vi "Proyecto.vi"() -> ()   [LabVIEW 2020]
uses:
  <vilib>/Utility/error.llb/DialogType.ctl
  <vilib>/Instr/_visa.llb/VISA Configure Serial Port (Instr).vi
panel:
  out "error out 2":errorcluster
  out "error out":errorcluster
  out "x+y":dbl
  out "Shape":i32
  out "B":i32
  out "G":i32
  out "R":i32
  out "Green object":dbl
  in  "ESP":bool
  in  "MATLAB":bool
  out "Position":i32
  out "Shape":picture
  out "Blue object":dbl
  out "Red object":dbl
  out "Color":u32(colorbox)
  out "Object presence":i32
  in  "Speed Control":dbl(slide) scale=80.0..100.0
  out "Band speed":dbl(knob) scale=0.0..10.0
  in  "ESP port":refnum<visa-resource-name>
  in  "Matlab port":refnum<visa-resource-name>
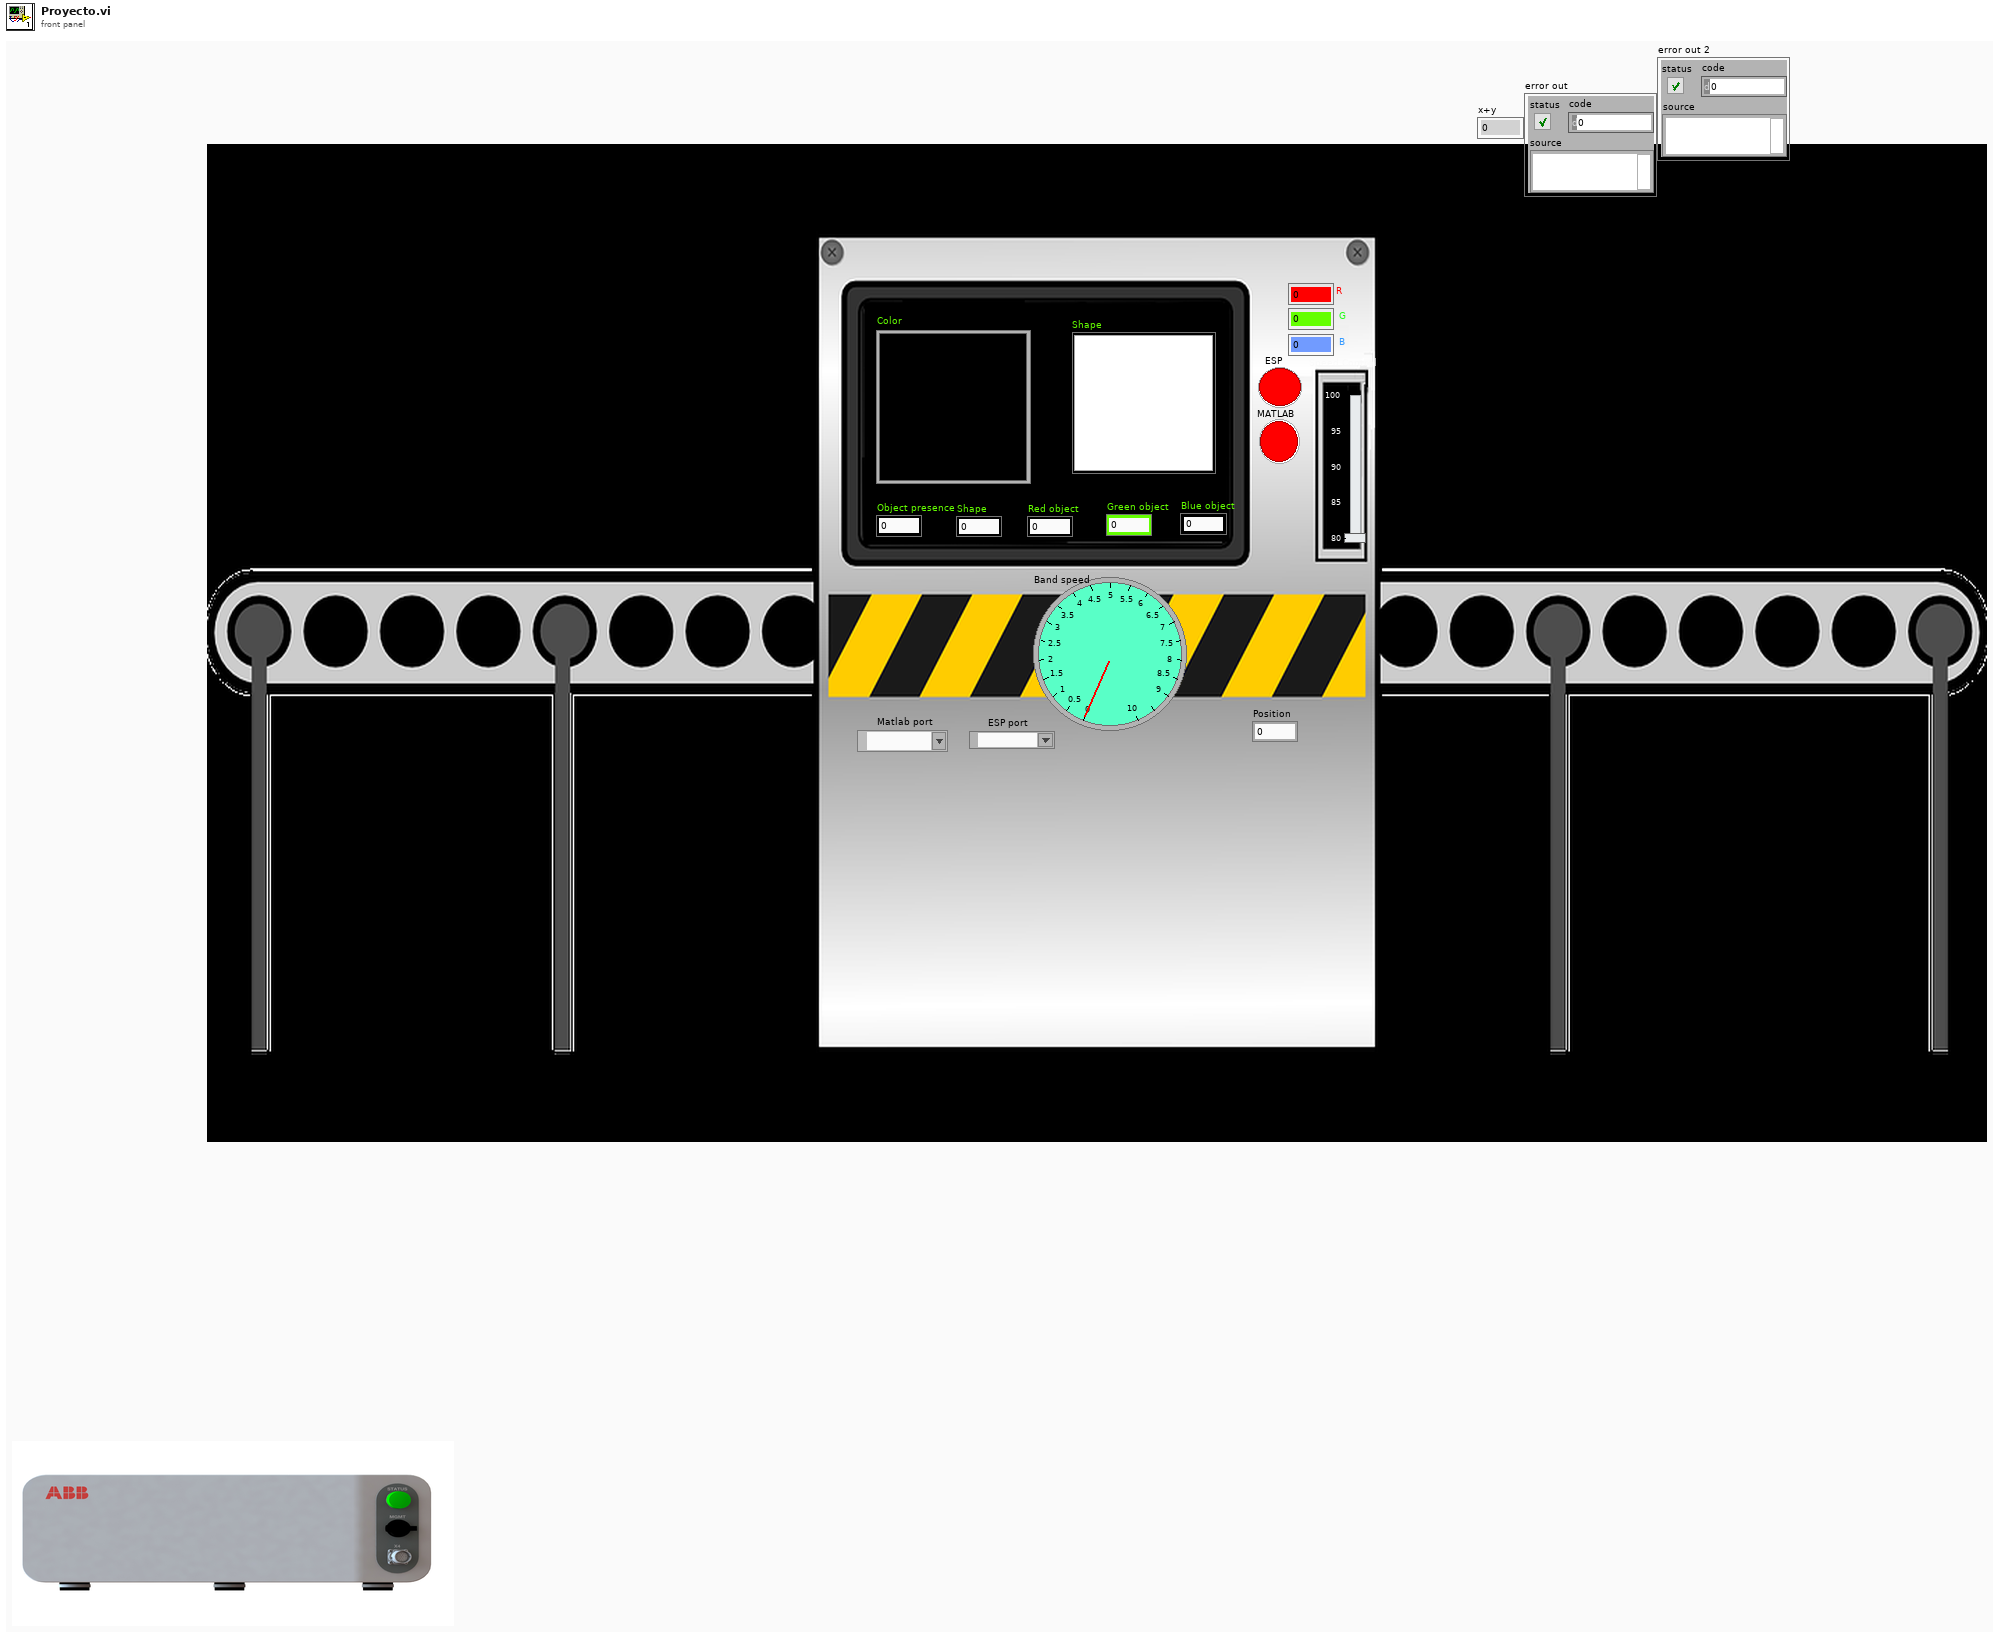
[diagram p1: front panel]
types:
  T1 = typedef "DialogType.ctl" = u16
  T2 = typedef "imagedata.ctl" = cluster{"image type":i32, "image depth":i32, "image":u8[], "mask":u8[], "colors":u32[], "Rectangle":cluster{"left":i16, "top":i16, "right":i16, "bottom":i16}}
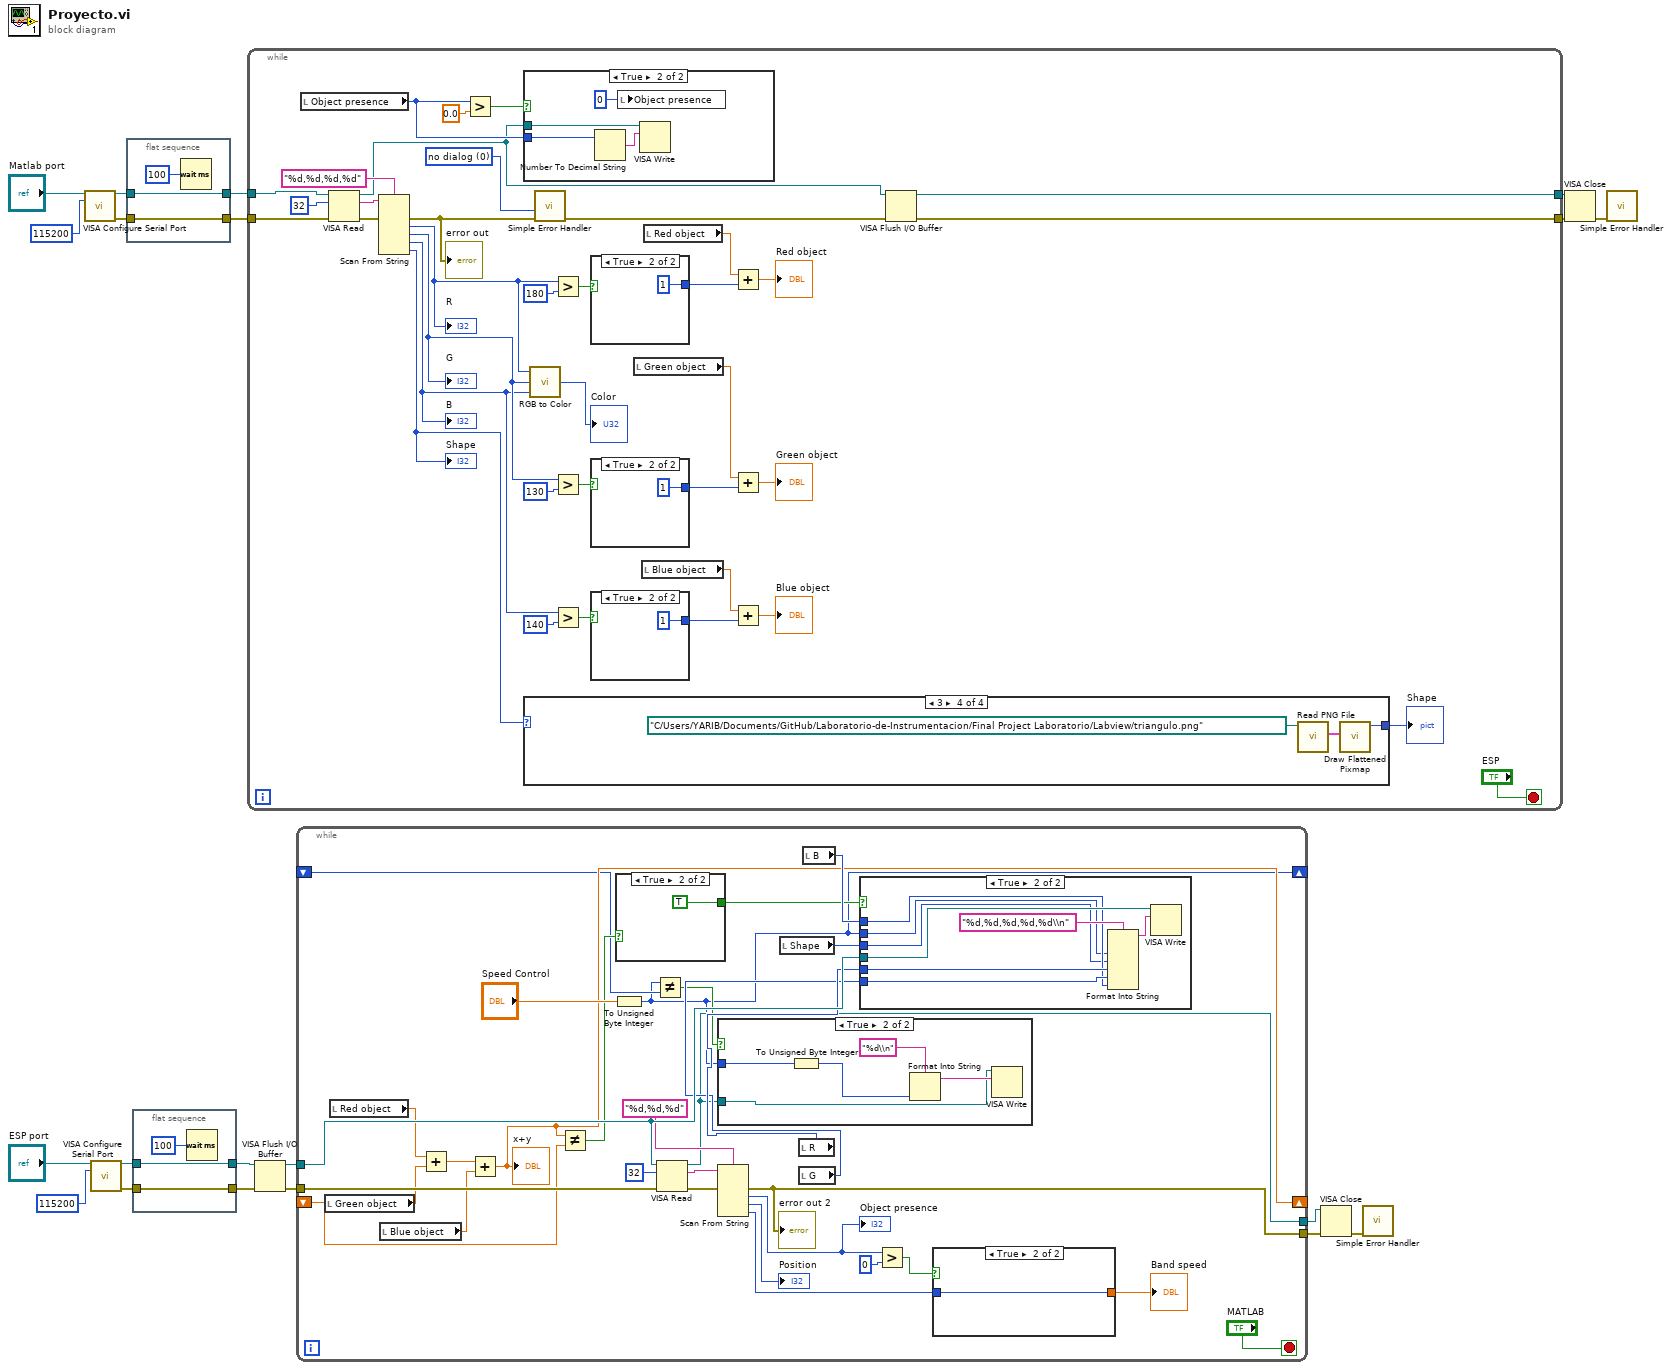
[diagram p0: block diagram]
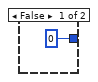
[diagram p2: hidden frame]
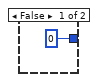
[diagram p4: hidden frame]
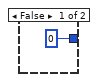
[diagram p5: hidden frame]
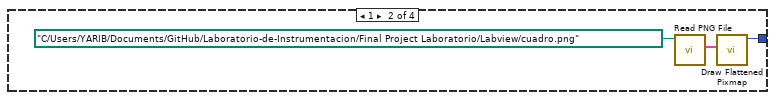
[diagram p7: hidden frame]
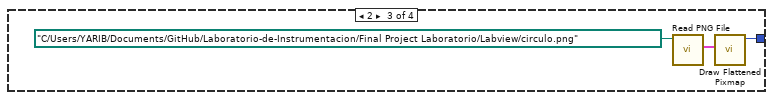
[diagram p8: hidden frame]
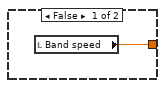
[diagram p9: hidden frame]
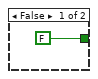
[diagram p11: hidden frame]
diagram:
  n1 = call-poly "VISA Configure Serial Port"("VISA resource name"="Matlab port", "baud rate (9600)"=u32 115200) -> ("VISA resource name out"=w10:refnum<visa-resource-name>, "error out"=w9:errorcluster)  [unwired: 12 in]
  n2 = call-poly "VISA Configure Serial Port"("VISA resource name"="ESP port", "baud rate (9600)"=u32 115200) -> ("VISA resource name out"=w3:refnum<visa-resource-name>, "error out"=w2:errorcluster)  [unwired: 12 in]
  n3 = flat-sequence {
    tunnel: w10 -> [w23]
    tunnel: [w23] -> w8
    tunnel: w9 -> [w22]
    tunnel: [w22] -> w7
    frame #0 {
      n4 = Wait (ms)(milliseconds to wait=u32 100) -> ()  [unwired: 1 out]
    }
  }
  n5 = flat-sequence {
    tunnel: w3 -> [w26]
    tunnel: w2 -> [w24]
    tunnel: [w26] -> w6
    tunnel: [w24] -> w1
    frame #0 {
      n6 = Wait (ms)(milliseconds to wait=u32 100) -> ()  [unwired: 1 out]
    }
  }
  n7 = while {
    tunnel: [w27] -> w13
    tunnel: [w28] -> w12
    tunnel: w8 -> [w33]
    tunnel: w7 -> [w32]
    stop <- "ESP" stop-if-true
    w54 = T1 0 items=["no dialog", "OK message", "continue or stop message", "OK message + warnings", "continue/stop + warnings"] ("type of dialog (OK msg:1)")
    n8 = local read "Object presence"() -> (w34:i32)
    n9 = VISA Read(VISA resource name=w33, byte count=u32 32, error in (no error)=w32) -> (VISA resource name out=w30:refnum<visa-resource-name>, read buffer=w56:string, error out=w57:errorcluster)  [unwired: 1 out]
    n10 = Scan From String(format string="%d,%d,%d,%d", input string=w56, error in=w57) -> (error out=w55:errorcluster, output 1=w46:i32, output 2=w48:i32, output 3=w47:i32, output 4=w49:i32)  [unwired: 5 in, 2 out]
    "R" <- w46
    "G" <- w48
    "B" <- w47
    "Shape" <- w49
    "error out" <- w55
    n11 = Greater?(x=w34, y=0.0) -> (0:w36:bool)
    n12 = case shown="True" w36 {
      tunnel: w30 -> [_ w69]
      tunnel: w34 -> [_ w68]
      frame False {
      }
      frame True {
        n13 = Number To Decimal String(number=w68) -> (decimal integer string=w67:string)  [unwired: 1 in]
        n14 = local write "Object presence"(0 ("Object presence")) -> ()
        n15 = VISA Write(VISA resource name=w69, write buffer=w67) -> ()  [unwired: 1 in, 3 out]
      }
    }
    n16 = case shown="3" w49 {
      tunnel: [_ w75 w78 w81] -> w60
      frame 0, Default {
      }
      frame 1 {
        n17 = call <vilib>:"Read PNG File.vi"("path to PNG file"=path "C:/Users/YARIB/Documents/GitHub/Laboratorio-de-Instrumentacion/Final Project Laboratorio/Labview/cuadro.png") -> ("image data"=w76:T2)  [unwired: 8 in, 2 out]
        n18 = call <vilib>:"Draw Flattened Pixmap.vi"("image data"=w76) -> ("new picture"=w75:picture)  [unwired: 8 in]
      }
      frame 2 {
        n19 = call <vilib>:"Read PNG File.vi"("path to PNG file"=path "C:/Users/YARIB/Documents/GitHub/Laboratorio-de-Instrumentacion/Final Project Laboratorio/Labview/circulo.png") -> ("image data"=w79:T2)  [unwired: 8 in, 2 out]
        n20 = call <vilib>:"Draw Flattened Pixmap.vi"("image data"=w79) -> ("new picture"=w78:picture)  [unwired: 8 in]
      }
      frame 3 {
        n21 = call <vilib>:"Read PNG File.vi"("path to PNG file"=path "C:/Users/YARIB/Documents/GitHub/Laboratorio-de-Instrumentacion/Final Project Laboratorio/Labview/triangulo.png") -> ("image data"=w82:T2)  [unwired: 8 in, 2 out]
        n22 = call <vilib>:"Draw Flattened Pixmap.vi"("image data"=w82) -> ("new picture"=w81:picture)  [unwired: 8 in]
      }
    }
    "Shape" <- w60
    n23 = call <vilib>:"RGB to Color.vi"("B"=w47, "G"=w48, "R"=w46) -> ("Color"=→"Color":u32)
    n24 = call <vilib>:"Simple Error Handler.vi"("type of dialog (OK msg:1)"=w54, "error in (no error)"=w55) -> ("error out"=w29:errorcluster)  [unwired: 3 in, 4 out]
    n25 = Greater?(x=w46, y=180) -> (0:w62:bool)
    n26 = Greater?(x=w48, y=130) -> (0:w53:bool)
    n27 = Greater?(x=w47, y=140) -> (0:w61:bool)
    n28 = case shown="True" w62 {
      tunnel: [0 1 ("y")] -> w42
      frame False {
      }
      frame True {
      }
    }
    n29 = case shown="True" w53 {
      tunnel: [0 1 ("y")] -> w45
      frame False {
      }
      frame True {
      }
    }
    n30 = case shown="True" w61 {
      tunnel: [0 1 ("y")] -> w39
      frame False {
      }
      frame True {
      }
    }
    n31 = local read "Green object"() -> (w43:dbl)
    n32 = local read "Blue object"() -> (w37:dbl)
    n33 = local read "Red object"() -> (w40:dbl)
    n34 = Add(x=w40, y=w42) -> (x+y=→"Red object":dbl)
    n35 = Add(x=w43, y=w45) -> (x+y=→"Green object":dbl)
    n36 = Add(x=w37, y=w39) -> (x+y=→"Blue object":dbl)
    n37 = VISA Flush I/O Buffer(VISA resource name=w30, error in (no error)=w29) -> (VISA resource name out=w27:refnum<visa-resource-name>, error out=w28:errorcluster)  [unwired: 1 in]
  }
  n38 = VISA Flush I/O Buffer(VISA resource name=w6, error in (no error)=w1) -> (VISA resource name out=w5:refnum<visa-resource-name>, error out=w4:errorcluster)  [unwired: 1 in]
  n39 = while {
    tunnel: w5 -> [w112]
    tunnel: [w90] -> w16
    tunnel: w4 -> [w113]
    tunnel: [w111] -> w17
    shift-right: [w94] -> _
    shift-left: _ -> [w93]
    shift-right: [w88] -> _
    shift-left: _ -> [w89]
    stop <- "MATLAB" stop-if-true
    n40 = local read "Green object"() -> (w100:dbl)
    n41 = local read "Red object"() -> (w99:dbl)
    n42 = local read "Blue object"() -> (w98:dbl)
    n43 = Add(x=w99, y=w100) -> (x+y=w101:dbl)
    n44 = Add(x=w101, y=w98) -> (x+y=w94:dbl)
    "x+y" <- w94
    n45 = Not Equal?(x=w94, y=w93) -> (x != y?=w95:bool)
    n46 = To Unsigned Byte Integer(number="Speed Control") -> (unsigned 8bit integer=w88:u8)
    n47 = case shown="True" w95 {
      tunnel: [FALSE TRUE] -> w97
      frame False {
      }
      frame True {
      }
    }
    n48 = Not Equal?(x=w88, y=w89) -> (x != y?=w91:bool)
    n49 = VISA Read(VISA resource name=w112, byte count=u32 32, error in (no error)=w113) -> (VISA resource name out=w90:refnum<visa-resource-name>, read buffer=w110:string, error out=w109:errorcluster)  [unwired: 1 out]
    n50 = case shown="True" w91 {
      tunnel: w90 -> [_ w116]
      tunnel: w88 -> [_ w117]
      frame False {
      }
      frame True {
        n51 = To Unsigned Byte Integer(number=w117) -> (unsigned 8bit integer=w120:u8)
        n52 = Format Into String(format string="%d\\n", w120) -> (resulting string=w118:string)  [unwired: 2 in, 1 out]
        n53 = VISA Write(VISA resource name=w116, write buffer=w118) -> ()  [unwired: 1 in, 3 out]
      }
    }
    n54 = Scan From String(format string="%d,%d,%d", input string=w110, error in=w109) -> (error out=w111:errorcluster, output 1=w86:i32, output 2=→"Position":i32, output 3=w83:i32)  [unwired: 4 in, 2 out]
    "Object presence" <- w86
    "error out 2" <- w111
    n55 = local read "Shape"() -> (w105:i32)
    n56 = local read "R"() -> (w104:i32)
    n57 = local read "G"() -> (w103:i32)
    n58 = local read "B"() -> (w102:i32)
    n59 = case shown="True" w97 {
      tunnel: w112 -> [_ w130]
      tunnel: w88 -> [_ w124]
      tunnel: w105 -> [_ w123]
      tunnel: w104 -> [_ w127]
      tunnel: w103 -> [_ w126]
      tunnel: w102 -> [_ w125]
      frame False {
      }
      frame True {
        n60 = Format Into String(format string="%d,%d,%d,%d,%d\\n", w124, w123, w127, w126, w125) -> (resulting string=w129:string)  [unwired: 2 in, 1 out]
        n61 = VISA Write(VISA resource name=w130, write buffer=w129) -> ()  [unwired: 1 in, 3 out]
      }
    }
    n62 = Greater?(x=w86, y=0) -> (0:w87:bool)
    n63 = case shown="True" w87 {
      tunnel: [w114 w115] -> w84
      tunnel: w83 -> [_ w115]
      frame False {
        n64 = local read "Band speed"() -> (w114:dbl)
      }
      frame True {
      }
    }
    "Band speed" <- w84
  }
  n65 = VISA Close(VISA resource name=w16, error in (no error)=w17) -> (error out=w18:errorcluster)
  n66 = call <vilib>:"Simple Error Handler.vi"("error in (no error)"=w18) -> ()  [unwired: 1 in, 8 out]
  n67 = VISA Close(VISA resource name=w13, error in (no error)=w12) -> (error out=w11:errorcluster)
  n68 = call <vilib>:"Simple Error Handler.vi"("error in (no error)"=w11) -> ()  [unwired: 1 in, 8 out]
